vi "Periodic Tasks.vi"(8 "error in":errorcluster) -> ()   [LabVIEW 2016]
doc: "This VI runs in parallel to other tasks. It can contain as many user-defined periodic loops as you need. These can carry out PID or other sorts of timed response."
uses:
  <vilib>/Rock Robotics/WPI/DriverStation/WPI_DriverStationRobotMode2.ctl
  Robot Global Data.vi
  <vilib>/Rock Robotics/Network Tables/NT Write Boolean.vi
  <vilib>/Rock Robotics/Network Tables/NT Write Number.vi
  <vilib>/Rock Robotics/Network Tables/NT Read String.vi
  <vilib>/Rock Robotics/Network Tables/NT Write String.vi
  <vilib>/Rock Robotics/Network Tables/NT Read Number.vi
  <vilib>/Rock Robotics/WPI/Utilities/WPI_GetSetVariantRefNum.vi
  <vilib>/Rock Robotics/Network Tables/NT Read Boolean.vi
  <vilib>/Rock Robotics/Network Tables/NT Write Numeric Array.vi
  <vilib>/Rock Robotics/Network Tables/NT Read Numeric Array.vi
panel:
  in  "milliseconds to wait":u32=20
  out "Averaged Values 2":dbl(graph)
  out "Channel 1":dbl(graph)
  out "Channel 0":dbl(graph)
  in  "Range":dbl=100.0 format="%#_13g"
  out "Averaged Values":dbl(graph)=25.833333333333332
  out "<5?":i16(graph)=1
  out "Image Width":dbl(graph)=26.0
  in  "Past array Width":dbl[](array[numeric])=[26.0, 26.0, 26.0, 25.0, 26.0, 26.0]
  out "Gear Orient":bool=TRUE
  out "Gear In":bool=TRUE
  out "1 Width":dbl=17.0
  out "1 Height":dbl=26.0
  out "2 Width":dbl=8.5
  out "2 Height":dbl=13.0
  in  "Past array":dbl[](array[numeric])=[-10.0, -10.0, -10.0]
  in  "Lcal Pixy Out":dbl=-10.0
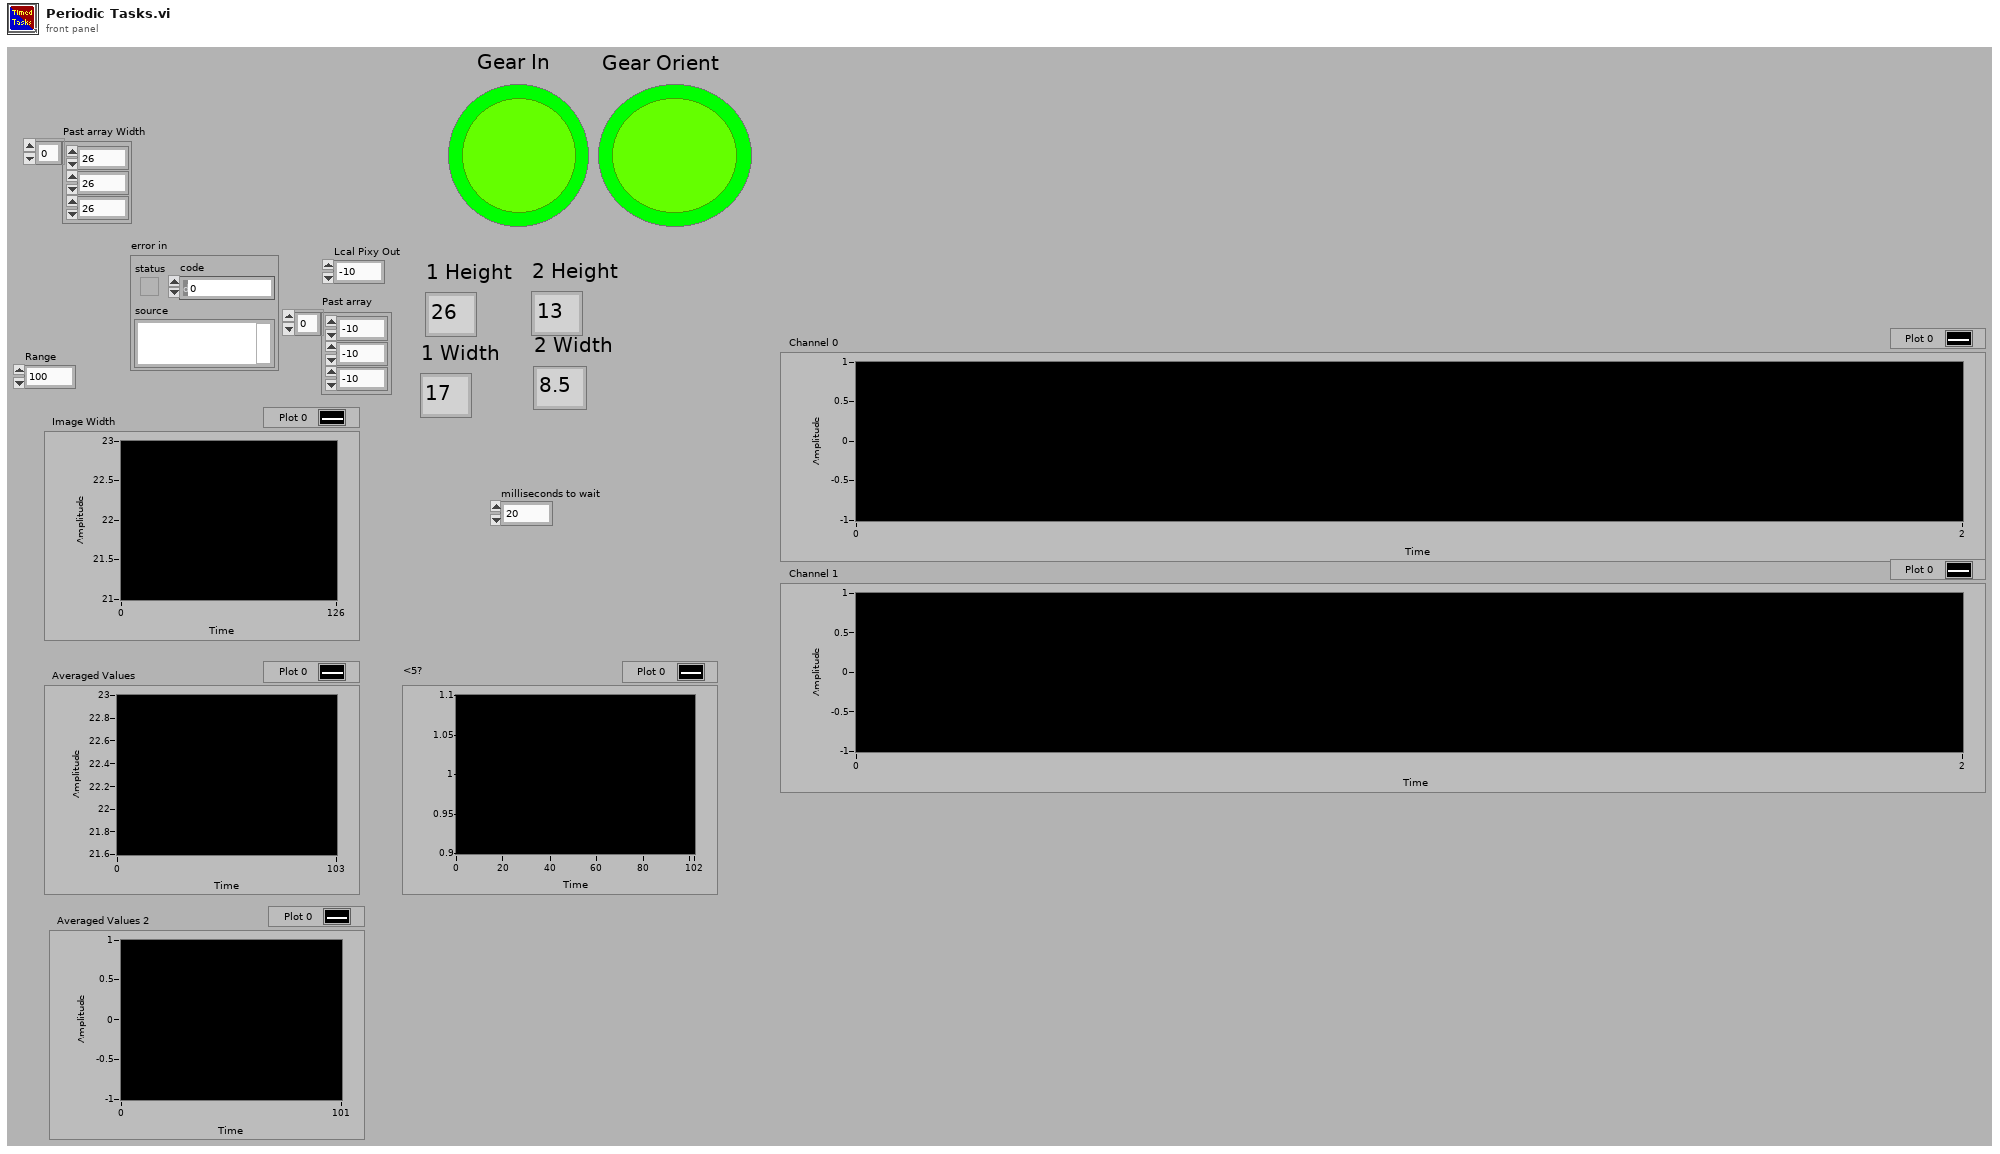
[diagram p1: front panel]
types:
  T1 = typedef "WPI_SwitchDevRef.ctl" = cluster{"DevStatus":errorcluster, "DIO Channel":T2, "CntIndex":T3, "Normally Closed":bool}
  T2 = typedef "FPGA_DIOChannel.ctl" = enum8{"DIO 0", "DIO 1", "DIO 2", "DIO 3", "DIO 4", "DIO 5", "DIO 6", "DIO 7", "DIO 8", "DIO 9", "DIO MXP 0", "DIO MXP 1", "DIO MXP 2", "DIO MXP 3", "DIO MXP 4", "DIO MXP 5", "DIO MXP 6", "DIO MXP 7", "DIO MXP 8", "DIO MXP 9", "DIO MXP 10", "DIO MXP 11", "DIO MXP 12", "DIO MXP 13", "DIO MXP 14", "DIO MXP 15", "SPI Port CS1", "SPI Port CS2", "SPI Port CS3", "SPI Port MISO", "SPI Port MOSI", "Invalid"}
  T3 = typedef "FPGA_CounterCtrSystemIndex.ctl" = enum8{"Ctr 0", "Ctr 1", "Ctr 2", "Ctr 3", "Ctr 4", "Ctr 5", "Ctr 6", "Ctr 7", "Invalid"}
  T4 = typedef "WPI_ServoDeviceRef.ctl" = cluster{"DeviceStatus":errorcluster, "PWM Channel":T5, "DeadBand":T6}
  T5 = typedef "FPGA_DIOPWMChannel.ctl" = enum8{"PWM 0", "PWM 1", "PWM 2", "PWM 3", "PWM 4", "PWM 5", "PWM 6", "PWM 7", "PWM 8", "PWM 9", "PWM MXP 0", "PWM MXP 1", "PWM MXP 2", "PWM MXP 3", "PWM MXP 4", "PWM MXP 5", "PWM MXP 6", "PWM MXP 7", "PWM MXP 8", "PWM MXP 9", "Invalid"}
  T6 = typedef "WPI_PWMDeadband.ctl" = cluster{"Name":string, "maxPositivePwm":i32, "minPositivePwm":i32, "centerPwm":i32, "maxNegativePwm":i32, "minNegativePwm":i32, "angularRange":u16}
  T7 = typedef "WPI_CounterDevRef.ctl" = cluster{"DevStatus":errorcluster, "CntIndex":T3}
  T8 = typedef "WPI_JoystickDevRef.ctl" = cluster{"Device":T9}
  T9 = typedef "WPI_JoystickDeviceEnum.ctl" = enum16{"USB 0", "USB 1", "USB 2", "USB 3", "USB 4", "USB 5"}
  T10 = typedef "WPI_DriverStationRobotMode2.ctl" = enum16{"Autonomous Disabled", "Autonomous Enabled", "Teleop Disabled", "Teleop Enabled", "Disconnected", "Finish", "Test Disabled", "Test Enabled", "Emergency Stopped"}
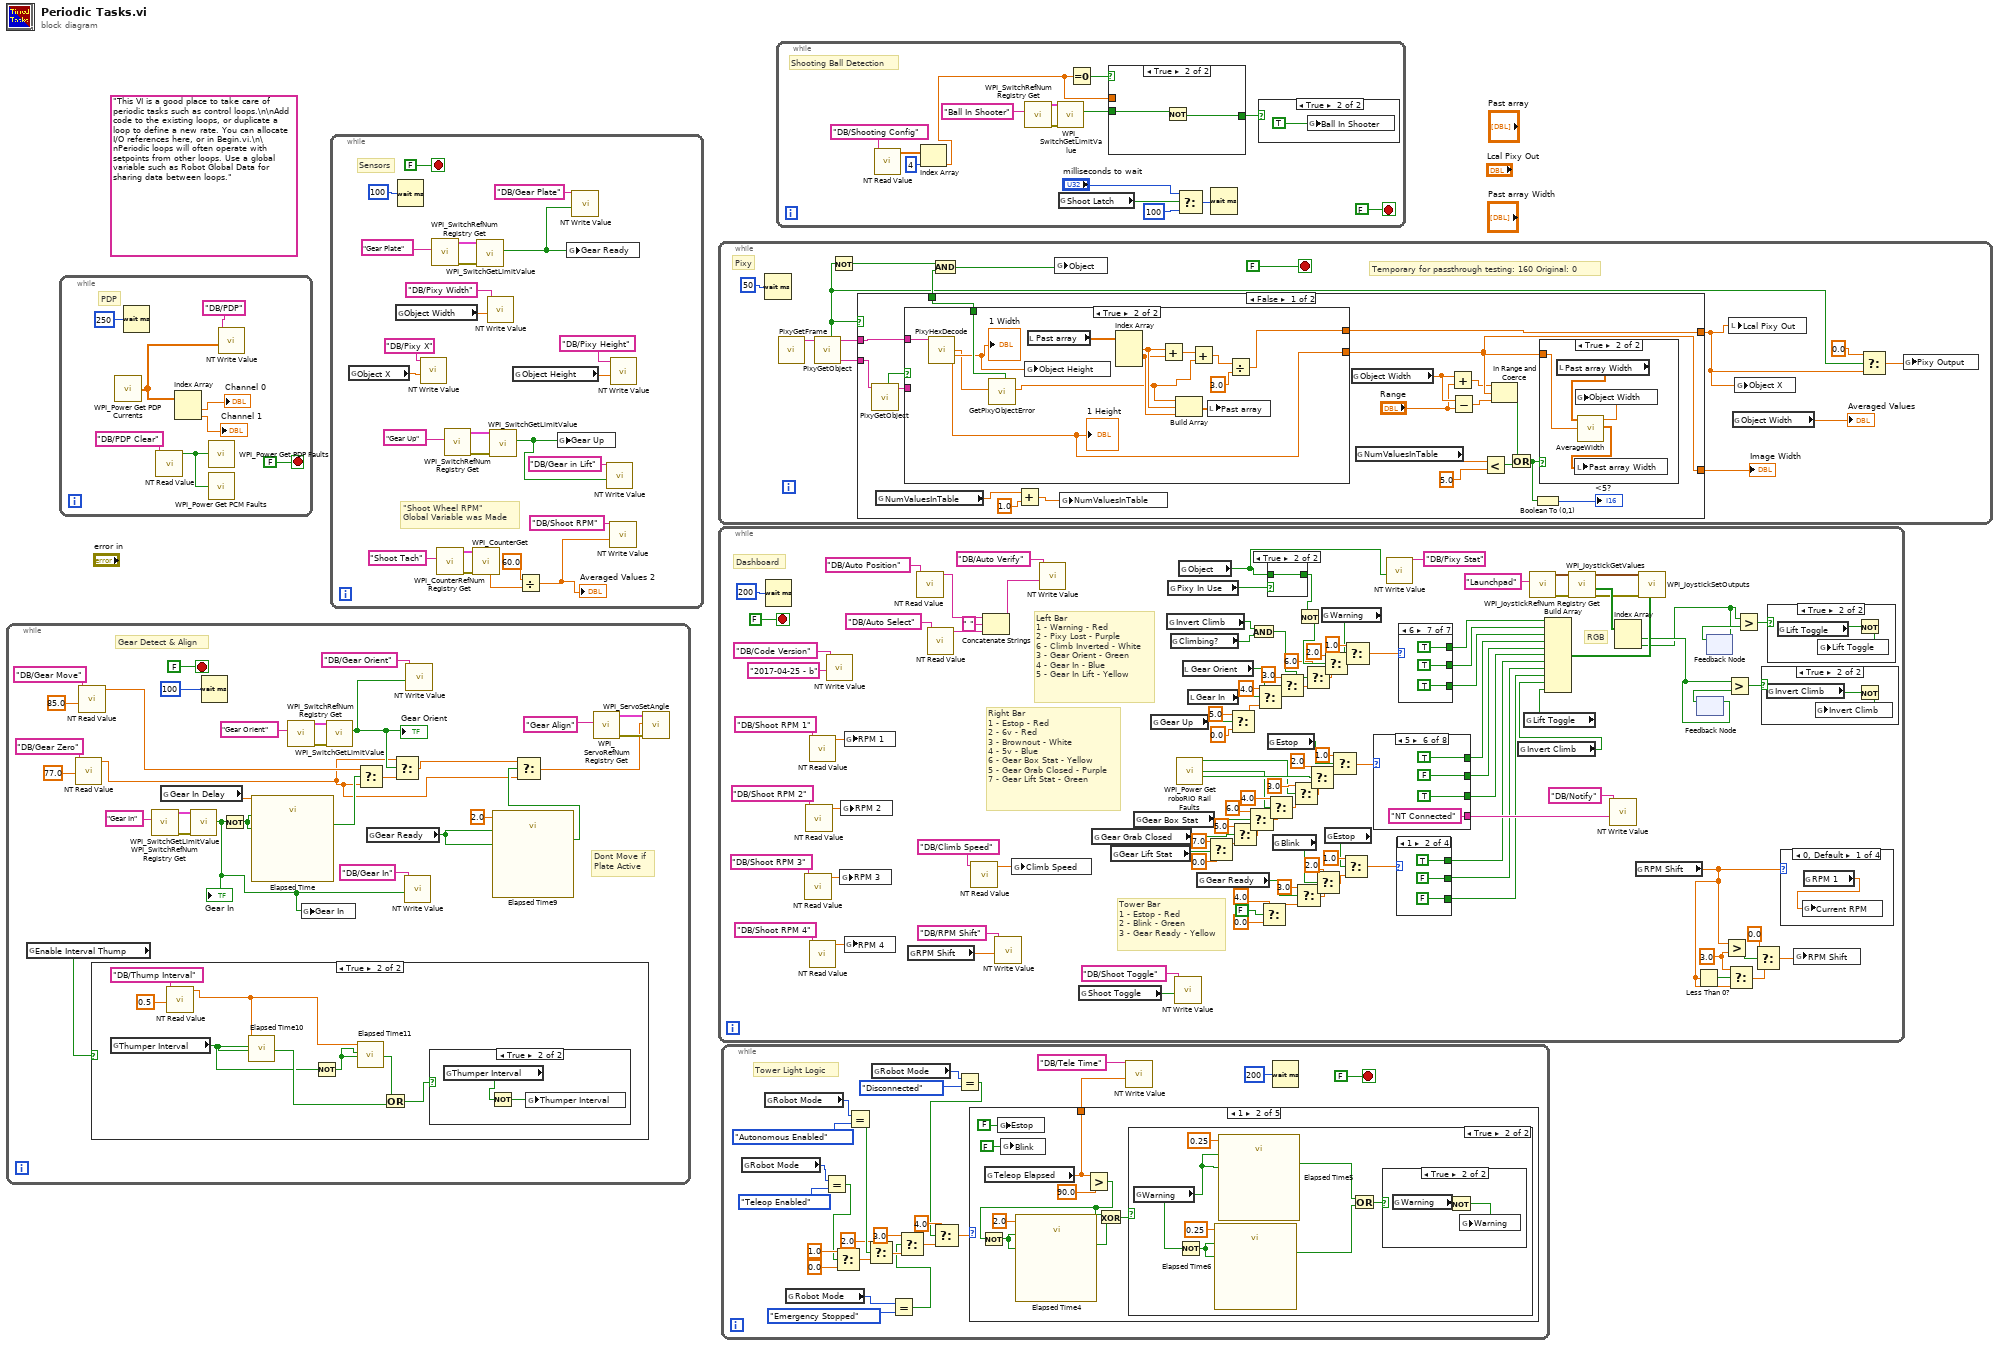
[diagram p0: block diagram]
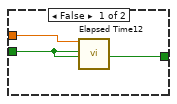
[diagram p2: hidden frame]
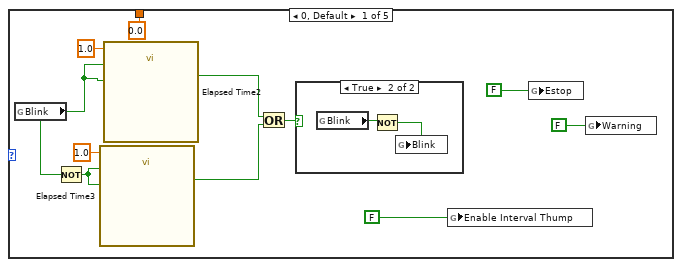
[diagram p4: hidden frame]
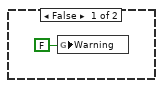
[diagram p6: hidden frame]
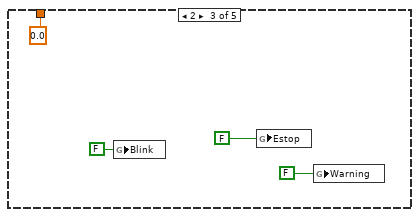
[diagram p8: hidden frame]
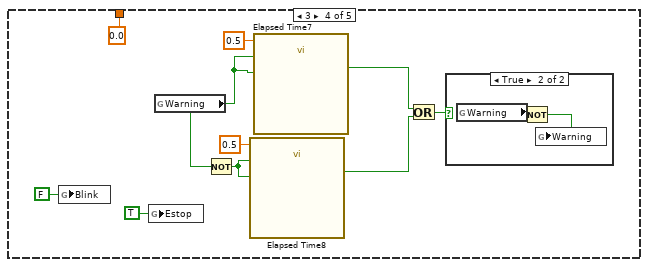
[diagram p9: hidden frame]
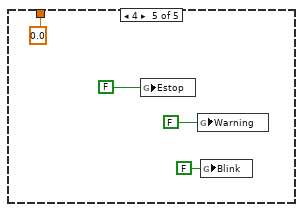
[diagram p11: hidden frame]
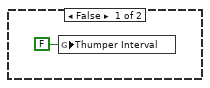
[diagram p12: hidden frame]
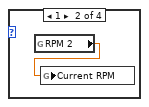
[diagram p14: hidden frame]
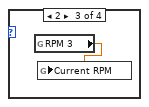
[diagram p15: hidden frame]
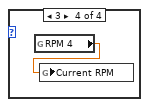
[diagram p16: hidden frame]
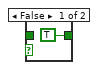
[diagram p19: hidden frame]
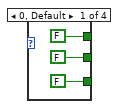
[diagram p20: hidden frame]
diagram:
  (unwired) "This VI is a good place to take care of periodic tasks such as control loops.\n\nAdd code to the existing loops, or duplicate a loop to define a new rate. You can allocate I/O references here, or in Begin.vi.\n\nPeriodic loops will often operate with setpoints from other loops. Use a global variable such as Robot Global Data for sharing data between loops."
  n1 = while {
    stop <- FALSE stop-if-true
    # "Dont Move if\nPlate Active"
    # "Gear Detect & Align"
    n2 = global read "Robot Global Data.vi" "Enable Interval Thump"() -> (w1:bool)
    n3 = call-poly <vilib>:"NT Read Value.vi"("Default Value"=77.0, "Name"="DB/Gear Zero") -> ("Numeric"=w3:dbl)  [unwired: 8 in, 1 out]
    n4 = call-poly <vilib>:"NT Read Value.vi"("Default Value"=85.0, "Name"="DB/Gear Move") -> ("Numeric"=w11:dbl)  [unwired: 8 in, 1 out]
    n5 = case shown="True" w1 {
      frame False {
        n6 = global write "Robot Global Data.vi" "Thumper Interval"(FALSE ("Thumper Interval")) -> ()
      }
      frame True {
        n7 = global read "Robot Global Data.vi" "Thumper Interval"() -> (w36:bool)
        n8 = call-poly <vilib>:"NT Read Value.vi"("Default Value"=0.5, "Name"="DB/Thump Interval") -> ("Numeric"=w33:dbl)  [unwired: 8 in, 1 out]
        n9 = call "Elapsed Time10"("Time Target (s)"=w33, "Reset"=w36, "Auto Reset"=w36) -> ("Time has Elapsed"=w38:bool)  [unwired: 9 in, 7 out]
        n10 = Not(x=w36) -> (.not. x?=w40:bool)
        n11 = call "Elapsed Time11"("Time Target (s)"=w33, "Reset"=w40, "Auto Reset"=w40) -> ("Time has Elapsed"=w39:bool)  [unwired: 9 in, 7 out]
        n12 = Or(x=w39, y=w38) -> (x .or. y?=w37:bool)
        n13 = case shown="True" w37 {
          frame False {
          }
          frame True {
            n14 = global read "Robot Global Data.vi" "Thumper Interval"() -> (w42:bool)
            n15 = Not(x=w42) -> (.not. x?=w41:bool)
            n16 = global write "Robot Global Data.vi" "Thumper Interval"(w41) -> ()
          }
        }
      }
    }
    n17 = call <vilib>:"WPI_SwitchRefNum Registry Get.vi"("refnum name"="Gear In") -> ("error out"=w28:errorcluster, "SwitchDevRef"=w29:T1)  [unwired: 9 in]
    n18 = global read "Robot Global Data.vi" "Gear In Delay"() -> (w21:dbl)
    n19 = call <vilib>:"WPI_SwitchGetLimitValue.vi"("error in (no error)"=w28, "SwitchDevRef"=w29) -> ("Switch Pressed"=w2:bool)  [unwired: 7 in, 2 out]
    "Gear In" <- w2
    n20 = Wait (ms)(milliseconds to wait=u32 100) -> ()  [unwired: 1 out]
    n21 = Not(x=w2) -> (.not. x?=w22:bool)
    n22 = call "Elapsed Time"("Time Target (s)"=w21, "Reset"=w22, "Auto Reset"=w22) -> ("Time has Elapsed"=w16:bool)  [unwired: 9 in, 7 out]
    n23 = call <vilib>:"WPI_SwitchRefNum Registry Get.vi"("refnum name"="Gear Orient") -> ("error out"=w24:errorcluster, "SwitchDevRef"=w25:T1)  [unwired: 9 in]
    n24 = global write "Robot Global Data.vi" "Gear In"(w2) -> ()
    n25 = call <vilib>:"WPI_SwitchGetLimitValue.vi"("error in (no error)"=w24, "SwitchDevRef"=w25) -> ("Switch Pressed"=w14:bool)  [unwired: 7 in, 2 out]
    "Gear Orient" <- w14
    n26 = Select(t=w11, s=w16, f=w3) -> (s? t:f=w26:dbl)
    n27 = global read "Robot Global Data.vi" "Gear Ready"() -> (w7:bool)
    n28 = Select(t=w3, s=w14, f=w26) -> (s? t:f=w4:dbl)
    n29 = call-poly <vilib>:"NT Write Value.vi"("Boolean"=w2, "Name"="DB/Gear In") -> ()  [unwired: 9 in, 1 out]
    n30 = call-poly <vilib>:"NT Write Value.vi"("Boolean"=w14, "Name"="DB/Gear Orient") -> ()  [unwired: 9 in, 1 out]
    n31 = call "Elapsed Time9"("Time Target (s)"=2.0, "Reset"=w7, "Auto Reset"=w7) -> ("Time has Elapsed"=w5:bool)  [unwired: 9 in, 7 out]
    n32 = Select(t=w4, s=w5, f=w3) -> (s? t:f=w8:dbl)
    n33 = call <vilib>:"WPI_ServoRefNum Registry Get.vi"("refnum name"="Gear Align") -> ("error out"=w17:errorcluster, "ServoDeviceRef"=w18:T4)  [unwired: 9 in]
    n34 = call <vilib>:"WPI_ServoSetAngle.vi"("error in (no error)"=w17, "Angle"=w8, "ServoDeviceRef"=w18) -> ()  [unwired: 7 in, 2 out]
  }
  n35 = while {
    stop <- FALSE stop-if-true
    # "PDP"
    n36 = call <vilib>:"WPI_Power Get PDP Currents.vi"() -> ("all currents (A)"=w45:dbl[])  [unwired: 13 in, 2 out]
    n37 = Wait (ms)(milliseconds to wait=u32 250) -> ()  [unwired: 1 out]
    n38 = call-poly <vilib>:"NT Read Value.vi"("Name"="DB/PDP Clear") -> ("Boolean"=w46:bool)  [unwired: 9 in, 1 out]
    n39 = Index Array(array=w45) -> (element #1=→"Channel 0":dbl, element #2=→"Channel 1":dbl)  [unwired: 2 in]
    n40 = call <vilib>:"WPI_Power Get PDP Faults.vi"("Clear Sticky Faults"=w46) -> ()  [unwired: 10 in, 5 out]
    n41 = call <vilib>:"WPI_Power Get PCM Faults.vi"("Clear Sticky Faults"=w46) -> ()  [unwired: 11 in, 4 out]
    n42 = call-poly <vilib>:"NT Write Value.vi"("Numeric Array"=w45, "Name"="DB/PDP") -> ()  [unwired: 9 in, 1 out]
  }
  n43 = while {
    stop <- FALSE stop-if-true
    # "\"Shoot Wheel RPM\"\nGlobal Variable was Made"
    # "Sensors"
    n44 = global read "Robot Global Data.vi" "Object X"() -> (w63:dbl)
    n45 = global read "Robot Global Data.vi" "Object Width"() -> (w65:dbl)
    n46 = Wait (ms)(milliseconds to wait=u32 100) -> ()  [unwired: 1 out]
    n47 = call-poly <vilib>:"NT Write Value.vi"("Numeric"=w63, "Name"="DB/Pixy X") -> ()  [unwired: 9 in, 1 out]
    n48 = call <vilib>:"WPI_SwitchRefNum Registry Get.vi"("refnum name"="Gear Plate") -> ("error out"=w73:errorcluster, "SwitchDevRef"=w72:T1)  [unwired: 9 in]
    n49 = call <vilib>:"WPI_CounterRefNum Registry Get.vi"("refnum name"="Shoot Tach") -> ("error out"=w54:errorcluster, "CounterDevRef"=w55:T7)  [unwired: 9 in]
    n50 = call <vilib>:"WPI_SwitchRefNum Registry Get.vi"("refnum name"="Gear Up") -> ("error out"=w62:errorcluster, "SwitchDevRef"=w61:T1)  [unwired: 9 in]
    n51 = call <vilib>:"WPI_CounterGet.vi"("error in (no error)"=w54, "CounterDevRef in"=w55) -> ("Period (sec)"=w57:dbl)  [unwired: 4 in, 5 out]
    n52 = call <vilib>:"WPI_SwitchGetLimitValue.vi"("error in (no error)"=w73, "SwitchDevRef"=w72) -> ("Switch Pressed"=w69:bool)  [unwired: 7 in, 2 out]
    n53 = call-poly <vilib>:"NT Write Value.vi"("Numeric"=w65, "Name"="DB/Pixy Width") -> ()  [unwired: 9 in, 1 out]
    n54 = call <vilib>:"WPI_SwitchGetLimitValue.vi"("error in (no error)"=w62, "SwitchDevRef"=w61) -> ("Switch Pressed"=w58:bool)  [unwired: 7 in, 2 out]
    n55 = global read "Robot Global Data.vi" "Object Height"() -> (w64:dbl)
    n56 = Divide(x=60.0, y=w57) -> (x/y=w51:dbl)
    "Averaged Values 2" <- w51
    n57 = global write "Robot Global Data.vi" "Gear Up"(w58) -> ()
    n58 = global write "Robot Global Data.vi" "Gear Ready"(w69) -> ()
    n59 = call-poly <vilib>:"NT Write Value.vi"("Boolean"=w69, "Name"="DB/Gear Plate") -> ()  [unwired: 9 in, 1 out]
    n60 = call-poly <vilib>:"NT Write Value.vi"("Boolean"=w58, "Name"="DB/Gear in Lift") -> ()  [unwired: 9 in, 1 out]
    n61 = call-poly <vilib>:"NT Write Value.vi"("Numeric"=w51, "Name"="DB/Shoot RPM") -> ()  [unwired: 9 in, 1 out]
    n62 = call-poly <vilib>:"NT Write Value.vi"("Numeric"=w64, "Name"="DB/Pixy Height") -> ()  [unwired: 9 in, 1 out]
  }
  n63 = while {
    stop <- FALSE stop-if-true
    # "Temporary for passthrough testing: 160 Original: 0"
    # "Pixy"
    n64 = Wait (ms)(milliseconds to wait=u32 50) -> ()  [unwired: 1 out]
    n65 = call "PixyGetFrame.vi"() -> ("Frame"=w84:string)  [unwired: 11 in]
    n66 = call "PixyGetObject.vi"("Input Frame"=w84) -> ("Remainder of Frame"=w83:string, "Object"=w82:string, "Empty?"=w80:bool)  [unwired: 8 in]
    n67 = Not(x=w80) -> (.not. x?=w86:bool)
    n68 = case shown="False" w80 {
      tunnel: [w109 w157] -> w78
      tunnel: w83 -> [w108 _]
      tunnel: w82 -> [w106 _]
      tunnel: [w104 FALSE] -> w81
      tunnel: [w98 w155] -> w77
      frame False {
        n69 = call "PixyGetObject.vi"("Input Frame"=w108) -> ("Object"=w105:string, "Empty?"=w107:bool)  [unwired: 8 in, 1 out]
        n70 = global read "Robot Global Data.vi" "NumValuesInTable"() -> (w101:dbl)
        n71 = case shown="True" w107 {
          tunnel: [w134 w148] -> w109
          tunnel: w106 -> [w130 w145]
          tunnel: w105 -> [w129 _]
          tunnel: [w126 w144] -> w104
          tunnel: [w114 w141] -> w98
          frame False {
            n72 = call "PixyHexDecode.vi"("Object"=w130) -> ("Y"=w116:dbl, "Width"=w119:dbl, "Height"=w121:dbl)  [unwired: 10 in, 2 out]
            n73 = call "PixyHexDecode.vi"("Object"=w129) -> ("Y"=w115:dbl, "Width"=w118:dbl, "Height"=w120:dbl)  [unwired: 10 in, 2 out]
            n74 = Add(x=w116, y=w115) -> (x+y=w132:dbl)
            n75 = Divide(x=w132, y=2.0) -> (x/y=w128:dbl)
            n76 = Add(x=w121, y=w120) -> (x+y=w125:dbl)
            n77 = local read "Past array"() -> (w140:dbl[])
            n78 = call "GetPixyObjectError.vi"("X Value"=w128) -> ("Output"=w127:dbl, "Object In Parameters"=w126:bool)  [unwired: 9 in]
            n79 = Divide(x=w125, y=2.0) -> (x/y=w114:dbl)
            "2 Height" <- w114
            n80 = Add(x=w119, y=w118) -> (x+y=w123:dbl)
            n81 = Index Array(array=w140) -> (element #1=w139:dbl, element #2=w138:dbl)  [unwired: 3 in, 1 out]
            n82 = Divide(x=w123, y=2.0) -> (x/y=w117:dbl)
            "2 Width" <- w117
            n83 = global write "Robot Global Data.vi" "Object Height"(w117) -> ()
            n84 = Add(x=w139, y=w138) -> (x+y=w137:dbl)
            n85 = Build Array(w127, w139, w138) -> (w133:dbl[])
            n86 = local write "Past array"(w133) -> ()
            n87 = Add(x=w137, y=w127) -> (x+y=w136:dbl)
            n88 = Divide(x=w136, y=3.0) -> (x/y=w134:dbl)
          }
          frame True {
            n89 = call "PixyHexDecode.vi"("Object"=w145) -> ("Y"=w142:dbl, "Width"=w143:dbl, "Height"=w141:dbl)  [unwired: 10 in, 2 out]
            "1 Width" <- w143
            "1 Height" <- w141
            n90 = call "GetPixyObjectError.vi"("X Value"=w142) -> ("Output"=w147:dbl, "Object In Parameters"=w144:bool)  [unwired: 9 in]
            n91 = global write "Robot Global Data.vi" "Object Height"(w143) -> ()
            n92 = local read "Past array"() -> (w154:dbl[])
            n93 = Index Array(array=w154) -> (element #1=w153:dbl, element #2=w152:dbl)  [unwired: 3 in, 1 out]
            n94 = Add(x=w153, y=w152) -> (x+y=w151:dbl)
            n95 = Build Array(w147, w153, w152) -> (w146:dbl[])
            n96 = Add(x=w151, y=w147) -> (x+y=w150:dbl)
            n97 = local write "Past array"(w146) -> ()
            n98 = Divide(x=w150, y=3.0) -> (x/y=w148:dbl)
          }
        }
        n99 = Add(x=w101, y=1.0) -> (x+y=w99:dbl)
        n100 = global write "Robot Global Data.vi" "NumValuesInTable"(w99) -> ()
        n101 = global read "Robot Global Data.vi" "Object Width"() -> (w97:dbl)
        n102 = global read "Robot Global Data.vi" "NumValuesInTable"() -> (w103:dbl)
        n103 = Add(x=w97, y="Range") -> (x+y=w94:dbl)
        n104 = Subtract(x=w97, y="Range") -> (x-y=w95:dbl)
        n105 = Less?(x=w103, y=5.0) -> (x < y?=w92:bool)
        n106 = In Range and Coerce(upper limit=w94, x=w98, lower limit=w95) -> (In Range?=w93:bool)  [unwired: 1 out]
        n107 = Or(x=w93, y=w92) -> (x .or. y?=w90:bool)
        n108 = Boolean To (0,1)(Boolean=w90) -> (0, 1=→"<5?":i16)
        n109 = case shown="True" w90 {
          tunnel: w98 -> [_ w112]
          frame False {
          }
          frame True {
            n110 = local read "Past array Width"() -> (w111:dbl[])
            n111 = call "AverageWidth.vi"("Width"=w112, "Past array Width"=w111) -> ("Array"=w110:dbl[], "mean"=w113:dbl)  [unwired: 8 in]
            n112 = local write "Past array Width"(w110) -> ()
            n113 = global write "Robot Global Data.vi" "Object Width"(w113) -> ()
          }
        }
      }
      frame True {
        w155 = 0.0 ("Height")
        n114 = local read "Lcal Pixy Out"() -> (w157:dbl)
        n115 = global write "Robot Global Data.vi" "NumValuesInTable"(w155) -> ()
      }
    }
    "Image Width" <- w77
    n116 = And(x=w86, y=w81) -> (x .and. y?=w85:bool)
    n117 = global write "Robot Global Data.vi" "Object"(w85) -> ()
    n118 = local write "Lcal Pixy Out"(w78) -> ()
    n119 = global read "Robot Global Data.vi" "Object Width"() -> (→"Averaged Values":dbl)
    n120 = global write "Robot Global Data.vi" "Object X"(w78) -> ()
    n121 = Select(t=0.0, s=w80, f=w78) -> (s? t:f=w79:dbl)
    n122 = global write "Robot Global Data.vi" "Pixy Output"(w79) -> ()
  }
  n123 = while {
    stop <- FALSE stop-if-true
    w184 = 3.0 ("y")
    # "Left Bar\n1 - Warning - Red\n2 - Pixy Lost - Purple \n6 - Climb Inverted - White\n3 - Gear Orient - Green\n4 - Gear In - Blue\n5 - Gear In Lift - Yellow"
    # "RGB"
    # "Tower Bar\n1 - Estop - Red\n2 - Blink - Green\n3 - Gear Ready - Yellow"
    # "Right Bar\n1 - Estop - Red\n2 - 6v - Red\n3 - Brownout - White\n4 - 5v - Blue\n6 - Gear Box Stat - Yellow\n5 - Gear Grab Closed - Purple\n7 - Gear Lift Stat - Green"
    # "Dashboard"
    n124 = Wait (ms)(milliseconds to wait=u32 200) -> ()  [unwired: 1 out]
    n125 = call-poly <vilib>:"NT Read Value.vi"("Name"="DB/Shoot RPM 3") -> ("Numeric"=w256:dbl)  [unwired: 9 in, 1 out]
    n126 = call-poly <vilib>:"NT Read Value.vi"("Name"="DB/Shoot RPM 2") -> ("Numeric"=w258:dbl)  [unwired: 9 in, 1 out]
    n127 = call-poly <vilib>:"NT Read Value.vi"("Name"="DB/Shoot RPM 1") -> ("Numeric"=w262:dbl)  [unwired: 9 in, 1 out]
    n128 = call-poly <vilib>:"NT Read Value.vi"("Name"="DB/Shoot RPM 4") -> ("Numeric"=w254:dbl)  [unwired: 9 in, 1 out]
    n129 = call-poly <vilib>:"NT Write Value.vi"("String"="2017-04-25 - b", "Name"="DB/Code Version") -> ()  [unwired: 9 in, 1 out]
    n130 = global write "Robot Global Data.vi" "RPM 3"(w256) -> ()
    n131 = global write "Robot Global Data.vi" "RPM 2"(w258) -> ()
    n132 = global write "Robot Global Data.vi" "RPM 1"(w262) -> ()
    n133 = global write "Robot Global Data.vi" "RPM 4"(w254) -> ()
    n134 = global read "Robot Global Data.vi" "RPM Shift"() -> (w252:dbl)
    n135 = call-poly <vilib>:"NT Read Value.vi"("Name"="DB/Auto Position") -> ("String"=w272:string)  [unwired: 9 in, 1 out]
    n136 = call-poly <vilib>:"NT Read Value.vi"("Name"="DB/Auto Select") -> ("String"=w273:string)  [unwired: 9 in, 1 out]
    n137 = call-poly <vilib>:"NT Read Value.vi"("Name"="DB/Climb Speed") -> ("Numeric"=w260:dbl)  [unwired: 9 in, 1 out]
    n138 = Concatenate Strings(w272, " " ("string"), w273) -> (w271:string)
    n139 = call-poly <vilib>:"NT Write Value.vi"("Numeric"=w252, "Name"="DB/RPM Shift") -> ()  [unwired: 9 in, 1 out]
    n140 = global write "Robot Global Data.vi" "Climb Speed"(w260) -> ()
    n141 = call-poly <vilib>:"NT Write Value.vi"("String"=w271, "Name"="DB/Auto Verify") -> ()  [unwired: 9 in, 1 out]
    n142 = global read "Robot Global Data.vi" "Shoot Toggle"() -> (w172:bool)
    n143 = global read "Robot Global Data.vi" "Gear Grab Closed"() -> (w165:bool)
    n144 = global read "Robot Global Data.vi" "Gear Lift Stat"() -> (w174:bool)
    n145 = global read "Robot Global Data.vi" "Gear Box Stat"() -> (w166:bool)
    n146 = global read "Robot Global Data.vi" "Gear Up"() -> (w169:bool)
    n147 = global read "Robot Global Data.vi" "Invert Climb"() -> (w160:bool)
    n148 = global read "Robot Global Data.vi" "Pixy In Use"() -> (w202:bool)
    n149 = global read "Robot Global Data.vi" "Climbing?"() -> (w159:bool)
    n150 = call-poly <vilib>:"NT Write Value.vi"("Boolean"=w172, "Name"="DB/Shoot Toggle") -> ()  [unwired: 9 in, 1 out]
    n151 = call <vilib>:"WPI_Power Get roboRIO Rail Faults.vi"() -> ("Input Voltage Brown Out"=w226:bool, "5 V User Rail Short"=w227:bool, "6 V User Rail Short"=w228:bool)  [unwired: 10 in, 3 out]
    n152 = global read "Robot Global Data.vi" "Object"() -> (w196:bool)
    n153 = local read "Gear Orient"() -> (w204:bool)
    n154 = local read "Gear In"() -> (w203:bool)
    n155 = global read "Robot Global Data.vi" "Gear Ready"() -> (w206:bool)
    n156 = Select(t=7.0, s=w174, f=0.0) -> (s? t:f=w177:dbl)
    n157 = Select(t=5.0, s=w169, f=0.0) -> (s? t:f=w170:dbl)
    n158 = Select(t=5.0, s=w165, f=w177) -> (s? t:f=w229:dbl)
    n159 = Select(t=6.0, s=w166, f=w229) -> (s? t:f=w230:dbl)
    n160 = And(x=w160, y=w159) -> (x .and. y?=w158:bool)
    n161 = Select(t=4.0, s=w203, f=w170) -> (s? t:f=w245:dbl)
    n162 = Select(t=4.0, s=FALSE, f=0.0) -> (s? t:f=w215:dbl)
    n163 = case shown="True" w202 {
      tunnel: [TRUE ("Object") w285] -> w200
      tunnel: w196 -> [_ w285]
      frame False {
      }
      frame True {
      }
    }
    n164 = global read "Robot Global Data.vi" "Estop"() -> (w232:bool)
    n165 = Select(t=4.0, s=w227, f=w230) -> (s? t:f=w237:dbl)
    n166 = global read "Robot Global Data.vi" "Blink"() -> (w207:bool)
    n167 = Select(t=3.0, s=w204, f=w245) -> (s? t:f=w161:dbl)
    n168 = Select(t=3.0, s=w226, f=w237) -> (s? t:f=w238:dbl)
    n169 = Select(t=3.0, s=w206, f=w215) -> (s? t:f=w216:dbl)
    n170 = Not(x=w200) -> (.not. x?=w201:bool)
    n171 = Select(t=6.0, s=w158, f=w161) -> (s? t:f=w163:dbl)
    n172 = Select(t=2.0, s=w228, f=w238) -> (s? t:f=w239:dbl)
    n173 = Select(t=2.0, s=w207, f=w216) -> (s? t:f=w217:dbl)
    n174 = global read "Robot Global Data.vi" "Warning"() -> (w219:bool)
    n175 = Select(t=2.0, s=w201, f=w163) -> (s? t:f=w249:dbl)
    n176 = global read "Robot Global Data.vi" "Estop"() -> (w208:bool)
    n177 = Select(t=1.0, s=w232, f=w239) -> (s? t:f=w233:dbl)
    n178 = Select(t=1.0, s=w208, f=w217) -> (s? t:f=w218:dbl)
    n179 = Select(t=1.0, s=w219, f=w249) -> (s? t:f=w250:dbl)
    n180 = case shown="5" w233 {
      tunnel: [FALSE TRUE TRUE TRUE FALSE TRUE TRUE FALSE] -> w222
      tunnel: [FALSE FALSE FALSE TRUE FALSE FALSE TRUE TRUE] -> w221
      tunnel: [FALSE FALSE FALSE TRUE TRUE TRUE FALSE FALSE] -> w220
      tunnel: ["NT Connected" ("String") "EStop - Reset Rio" ("String") "6v Rail Short" ("String") "Brownout" ("String") "5v Rail Short" ("String") "NT Connected" ("String") "NT Connected" ("String") "NT Connected" ("String")] -> w240
      frame 0, Default {
      }
      frame 1 {
      }
      frame 2 {
      }
      frame 3 {
      }
      frame 4 {
      }
      frame 5 {
      }
      frame 6 {
      }
      frame 7 {
      }
    }
    n181 = call-poly <vilib>:"NT Write Value.vi"("Boolean"=w196, "Name"="DB/Pixy Stat") -> ()  [unwired: 9 in, 1 out]
    n182 = case shown="1" w218 {
      tunnel: [FALSE TRUE FALSE TRUE] -> w199
      tunnel: [FALSE FALSE TRUE TRUE] -> w198
      tunnel: [FALSE FALSE FALSE FALSE] -> w197
      frame 0, Default {
      }
      frame 1 {
      }
      frame 2 {
      }
      frame 3 {
      }
    }
    n183 = case shown="6" w250 {
      tunnel: [FALSE TRUE TRUE FALSE FALSE TRUE TRUE] -> w248
      tunnel: [FALSE FALSE FALSE TRUE FALSE TRUE TRUE] -> w247
      tunnel: [FALSE FALSE TRUE FALSE TRUE FALSE TRUE] -> w246
      frame 0, Default {
      }
      frame 1 {
      }
      frame 2 {
      }
      frame 3 {
      }
      frame 4 {
      }
      frame 5 {
      }
      frame 6 {
      }
    }
    n184 = global read "Robot Global Data.vi" "Invert Climb"() -> (w164:bool)
    n185 = global read "Robot Global Data.vi" "Lift Toggle"() -> (w171:bool)
    n186 = call <vilib>:"WPI_JoystickRefNum Registry Get.vi"("refnum name"="Launchpad") -> ("error out"=w183:errorcluster, "JoystickDevRef"=w182:T8)  [unwired: 9 in]
    n187 = Build Array(w248, w247, w246, w222, w221, w220, w199, w198, w197, w164, w171) -> (w223:bool[])
    n188 = call <vilib>:"WPI_JoystickGetValues.vi"("error in (no error)"=w183, "JoystickDevRef"=w182) -> ("error out"=w180:errorcluster, "Buttons"=w195:bool[], "JoystickDevRef"=w181:T8)  [unwired: 5 in, 2 out]
    n189 = call-poly <vilib>:"NT Write Value.vi"("String"=w240, "Name"="DB/Notify") -> ()  [unwired: 9 in, 1 out]
    n190 = Index Array(array=w195) -> (element #1=w179:bool, element #2=w178:bool)  [unwired: 2 in]
    n191 = global read "Robot Global Data.vi" "RPM Shift"() -> (w185:dbl)
    n192 = call <vilib>:"WPI_JoystickSetOutputs.vi"("Outputs"=w223, "error in (no error)"=w180, "JoystickDevRef"=w181) -> ()  [unwired: 7 in, 2 out]
    n193 = Less Than 0?(x=w185) -> (x < 0?=w188:bool)
    n194 = feedback #1() -> (w191:bool)  [unwired: 1 in]
    n195 = feedback-in #1(w179) -> ()
    n196 = feedback #2() -> (w193:bool)  [unwired: 1 in]
    n197 = feedback-in #2(w178) -> ()
    n198 = Greater?(x=w185, y=w184) -> (0:w187:bool)
    n199 = Greater?(x=w179, y=w191) -> (0:w192:bool)
    n200 = Select(t=w184, s=w188, f=w185) -> (s? t:f=w189:dbl)
    n201 = Greater?(x=w178, y=w193) -> (0:w194:bool)
    n202 = Select(t=0.0, s=w187, f=w189) -> (s? t:f=w190:dbl)
    n203 = case shown="True" w192 {
      frame False {
      }
      frame True {
        n204 = global read "Robot Global Data.vi" "Invert Climb"() -> (w281:bool)
        n205 = Not(x=w281) -> (.not. x?=w280:bool)
        n206 = global write "Robot Global Data.vi" "Invert Climb"(w280) -> ()
      }
    }
    n207 = case shown="True" w194 {
      frame False {
      }
      frame True {
        n208 = global read "Robot Global Data.vi" "Lift Toggle"() -> (w283:bool)
        n209 = Not(x=w283) -> (.not. x?=w282:bool)
        n210 = global write "Robot Global Data.vi" "Lift Toggle"(w282) -> ()
      }
    }
    n211 = case shown="0, Default" w185 {
      frame 0, Default {
        n212 = global read "Robot Global Data.vi" "RPM 1"() -> (w276:dbl)
        n213 = global write "Robot Global Data.vi" "Current RPM"(w276) -> ()
      }
      frame 1 {
        n214 = global read "Robot Global Data.vi" "RPM 2"() -> (w277:dbl)
        n215 = global write "Robot Global Data.vi" "Current RPM"(w277) -> ()
      }
      frame 2 {
        n216 = global read "Robot Global Data.vi" "RPM 3"() -> (w278:dbl)
        n217 = global write "Robot Global Data.vi" "Current RPM"(w278) -> ()
      }
      frame 3 {
        n218 = global read "Robot Global Data.vi" "RPM 4"() -> (w279:dbl)
        n219 = global write "Robot Global Data.vi" "Current RPM"(w279) -> ()
      }
    }
    n220 = global write "Robot Global Data.vi" "RPM Shift"(w190) -> ()
  }
  n221 = while {
    stop <- FALSE stop-if-true
    # "Tower Light Logic"
    n222 = global read "Robot Global Data.vi" "Robot Mode"() -> (w372:T10)
    n223 = global read "Robot Global Data.vi" "Robot Mode"() -> (w366:T10)
    n224 = global read "Robot Global Data.vi" "Robot Mode"() -> (w374:T10)
    n225 = Equal?(x=w372, y=WPI_DriverStationRobotMode2."Teleop Enabled") -> (x = y?=w362:bool)
    n226 = Select(t=1.0, s=w362, f=0.0) -> (s? t:f=w369:dbl)
    n227 = Equal?(x=w366, y=WPI_DriverStationRobotMode2."Autonomous Enabled") -> (x = y?=w364:bool)
    n228 = Select(t=2.0, s=w364, f=w369) -> (s? t:f=w361:dbl)
    n229 = global read "Robot Global Data.vi" "Robot Mode"() -> (w357:T10)
    n230 = Equal?(x=w374, y=WPI_DriverStationRobotMode2."Emergency Stopped") -> (x = y?=w358:bool)
    n231 = Select(t=3.0, s=w358, f=w361) -> (s? t:f=w359:dbl)
    n232 = Equal?(x=w357, y=WPI_DriverStationRobotMode2."Disconnected") -> (x = y?=w354:bool)
    n233 = Select(t=4.0, s=w354, f=w359) -> (s? t:f=w353:dbl)
    n234 = case shown="1" w353 {
      tunnel: [0.0 ("Teleop Elapsed") w389 0.0 ("Teleop Elapsed") 0.0 ("Teleop Elapsed") 0.0 ("Teleop Elapsed")] -> w351
      frame 0, Default {
        n235 = global read "Robot Global Data.vi" "Blink"() -> (w380:bool)
        n236 = Not(x=w380) -> (.not. x?=w381:bool)
        n237 = call "Elapsed Time3"("Time Target (s)"=1.0, "Reset"=w381, "Auto Reset"=w381) -> ("Time has Elapsed"=w382:bool)  [unwired: 9 in, 7 out]
        n238 = call "Elapsed Time2"("Time Target (s)"=1.0, "Reset"=w380, "Auto Reset"=w380) -> ("Time has Elapsed"=w383:bool)  [unwired: 9 in, 7 out]
        n239 = Or(x=w383, y=w382) -> (x .or. y?=w384:bool)
        n240 = case shown="True" w384 {
          frame False {
          }
          frame True {
            n241 = global read "Robot Global Data.vi" "Blink"() -> (w388:bool)
            n242 = Not(x=w388) -> (.not. x?=w387:bool)
            n243 = global write "Robot Global Data.vi" "Blink"(w387) -> ()
          }
        }
        n244 = global write "Robot Global Data.vi" "Enable Interval Thump"(FALSE) -> ()
        n245 = global write "Robot Global Data.vi" "Estop"(FALSE ("Blink")) -> ()
        n246 = global write "Robot Global Data.vi" "Warning"(FALSE ("Blink")) -> ()
      }
      frame 1 {
        n247 = global read "Robot Global Data.vi" "Teleop Elapsed"() -> (w389:dbl)
        n248 = global write "Robot Global Data.vi" "Estop"(FALSE ("Blink")) -> ()
        n249 = global write "Robot Global Data.vi" "Blink"(FALSE ("Blink")) -> ()
        n250 = Greater?(x=w389, y=90.0) -> (0:w393:bool)
        n251 = Not(x=w393) -> (.not. x?=w396:bool)
        n252 = call "Elapsed Time4"("Time Target (s)"=2.0, "Reset"=w396, "Auto Reset"=w396) -> ("Time has Elapsed"=w391:bool)  [unwired: 9 in, 7 out]
        n253 = Exclusive Or(1:w391, 2:w393) -> (0:w392:bool)
        n254 = case shown="True" w392 {
          frame False {
            n255 = global write "Robot Global Data.vi" "Warning"(FALSE ("Blink")) -> ()
          }
          frame True {
            n256 = global read "Robot Global Data.vi" "Warning"() -> (w399:bool)
            n257 = Not(x=w399) -> (.not. x?=w400:bool)
            n258 = call "Elapsed Time6"("Time Target (s)"=0.25, "Reset"=w400, "Auto Reset"=w400) -> ("Time has Elapsed"=w401:bool)  [unwired: 9 in, 7 out]
            n259 = call "Elapsed Time5"("Time Target (s)"=0.25, "Reset"=w399, "Auto Reset"=w399) -> ("Time has Elapsed"=w402:bool)  [unwired: 9 in, 7 out]
            n260 = Or(x=w402, y=w401) -> (x .or. y?=w403:bool)
            n261 = case shown="True" w403 {
              frame False {
              }
              frame True {
                n262 = global read "Robot Global Data.vi" "Warning"() -> (w407:bool)
                n263 = Not(x=w407) -> (.not. x?=w406:bool)
                n264 = global write "Robot Global Data.vi" "Warning"(w406) -> ()
              }
            }
          }
        }
      }
      frame 2 {
        n265 = global write "Robot Global Data.vi" "Blink"(FALSE ("Blink")) -> ()
        n266 = global write "Robot Global Data.vi" "Estop"(FALSE ("Blink")) -> ()
        n267 = global write "Robot Global Data.vi" "Warning"(FALSE ("Blink")) -> ()
      }
      frame 3 {
        n268 = global write "Robot Global Data.vi" "Blink"(FALSE ("Blink")) -> ()
        n269 = global write "Robot Global Data.vi" "Estop"(TRUE ("Estop")) -> ()
        n270 = global read "Robot Global Data.vi" "Warning"() -> (w414:bool)
        n271 = Not(x=w414) -> (.not. x?=w416:bool)
        n272 = call "Elapsed Time8"("Time Target (s)"=0.5, "Reset"=w416, "Auto Reset"=w416) -> ("Time has Elapsed"=w417:bool)  [unwired: 9 in, 7 out]
        n273 = call "Elapsed Time7"("Time Target (s)"=0.5, "Reset"=w414, "Auto Reset"=w414) -> ("Time has Elapsed"=w418:bool)  [unwired: 9 in, 7 out]
        n274 = Or(x=w418, y=w417) -> (x .or. y?=w419:bool)
        n275 = case shown="True" w419 {
          frame False {
          }
          frame True {
            n276 = global read "Robot Global Data.vi" "Warning"() -> (w423:bool)
            n277 = Not(x=w423) -> (.not. x?=w422:bool)
            n278 = global write "Robot Global Data.vi" "Warning"(w422) -> ()
          }
        }
      }
      frame 4 {
        n279 = global write "Robot Global Data.vi" "Estop"(FALSE ("Blink")) -> ()
        n280 = global write "Robot Global Data.vi" "Warning"(FALSE ("Blink")) -> ()
        n281 = global write "Robot Global Data.vi" "Blink"(FALSE ("Blink")) -> ()
      }
    }
    n282 = call-poly <vilib>:"NT Write Value.vi"("Numeric"=w351, "Name"="DB/Tele Time") -> ()  [unwired: 9 in, 1 out]
    n283 = Wait (ms)(milliseconds to wait=u32 200) -> ()  [unwired: 1 out]
  }
  n284 = while {
    stop <- FALSE stop-if-true
    # "Shooting Ball Detection"
    n285 = call-poly <vilib>:"NT Read Value.vi"("Name"="DB/Shooting Config") -> ("Numeric Array"=w436:dbl[])  [unwired: 9 in, 1 out]
    n286 = Index Array(array=w436, index=4) -> (element=w429:dbl)
    n287 = call <vilib>:"WPI_SwitchRefNum Registry Get.vi"("refnum name"="Ball In Shooter") -> ("error out"=w433:errorcluster, "SwitchDevRef"=w432:T1)  [unwired: 9 in]
    n288 = call <vilib>:"WPI_SwitchGetLimitValue.vi"("error in (no error)"=w433, "SwitchDevRef"=w432) -> ("Switch Pressed"=w428:bool)  [unwired: 7 in, 2 out]
    n289 = global read "Robot Global Data.vi" "Shoot Latch"() -> (w438:bool)
    n290 = Equal To 0?(x=w429) -> (x = 0?=w430:bool)
    n291 = case shown="True" w430 {
      tunnel: w428 -> [w445 w447]
      tunnel: [w444 w446] -> w431
      tunnel: w429 -> [w443 _]
      frame False {
        n292 = call "Elapsed Time12"("Time Target (s)"=w443, "Reset"=w445, "Auto Reset"=w445) -> ("Time has Elapsed"=w444:bool)  [unwired: 9 in, 7 out]
      }
      frame True {
        n293 = Not(x=w447) -> (.not. x?=w446:bool)
      }
    }
    n294 = Select(t="milliseconds to wait", s=w438, f=u32 100) -> (s? t:f=w440:u32)
    n295 = Wait (ms)(milliseconds to wait=w440) -> ()  [unwired: 1 out]
    n296 = case shown="True" w431 {
      frame False {
      }
      frame True {
        n297 = global write "Robot Global Data.vi" "Ball In Shooter"(TRUE) -> ()
      }
    }
  }
